vi "Rename Plugin Data File.vi"(0 "configuration":T1, 5 "plugin library path":path, 11 "error in":errorcluster) -> (4 "plugin data file path":path, 15 "error out":errorcluster)   [LabVIEW 2021, in "InstrumentStudio Plug-In Editor.lvlib"]
uses:
  InstrumentStudio Plug-In Editor.lvlib
  Data Holder.ctl
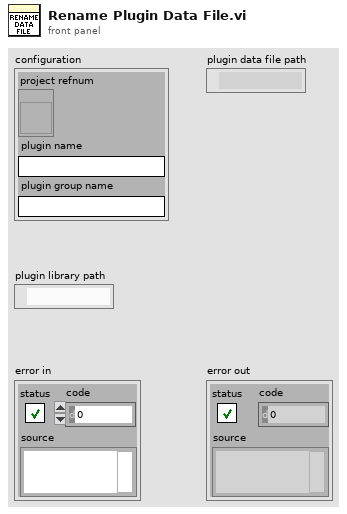
[diagram p1: front panel]
types:
  T1 = typedef "InstrumentStudio Plug-In Editor.lvlib/Data Holder.ctl" = cluster{"project refnum":refnum<vi>, "plugin name":string, "plugin group name":string}
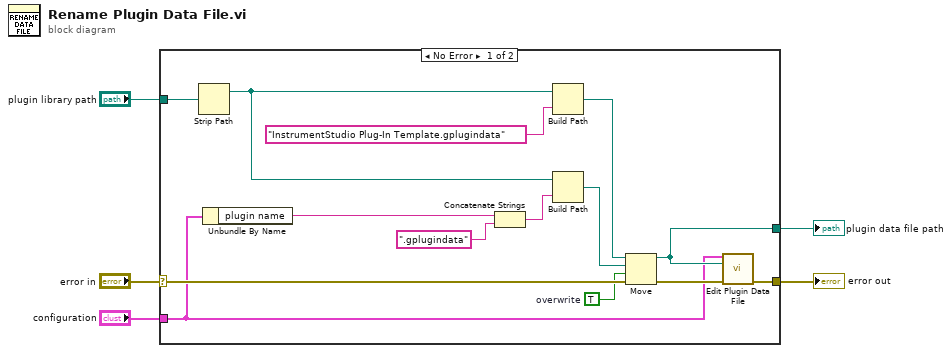
[diagram p0: block diagram]
diagram:
  n1 = case shown="No Error" "error in" {
    selector: "error in" -> [w19 w20]
    tunnel: [w17 w20] -> w5
    tunnel: "configuration" -> [w11 _]
    tunnel: [w12 _] -> w4
    tunnel: "plugin library path" -> [w8 _]
    frame No Error {
      w13 = TRUE  # overwrite
      n2 = Strip Path(path=w8) -> (stripped path=w6:path)  [unwired: 1 out]
      n3 = Unbundle By Name(w11) -> ("plugin name"=w16:string)
      n4 = Concatenate Strings(w16, ".gplugindata" ("string")) -> (w7:string)
      n5 = Build Path(base path=w6, name or relative path="InstrumentStudio Plug-In Template.gplugindata" ("string")) -> (appended path=w15:path)
      n6 = Build Path(base path=w6, name or relative path=w7) -> (appended path=w14:path)
      n7 = Move(source path=w15, error in=w19, 9:w13, 10:w14) -> (error out=w18:errorcluster, 3:w12:path)  [unwired: 1 in, 1 out]
      n8 = call "Edit Plugin Data File.vi"("configuration"=w11, "plugin data file path"=w12, "error in"=w18) -> ("error out"=w17:errorcluster)  [unwired: 12 in]
    }
    frame Error {
    }
  }
  "error out" <- w5
  "plugin data file path" <- w4
